vi "Write To Report.vi"(8 "error in (no error)":errorcluster, 11 "Report Info":T1[](array[typedef])) -> (0 "error out":errorcluster)   [LabVIEW 2018, in "File IO.lvlib"]
doc: "This subVI enqueues the named action in to the communications queue along with the input data."
uses:
  File IO.lvlib
  Private Controls/Module Action.ctl
  Public Controls/Write to Report.ctl
  Public Controls/Report Sheet Names.ctl
  Private Controls/Module Data.ctl
panel:
  in  "Action":T3=enum."Write To Report"
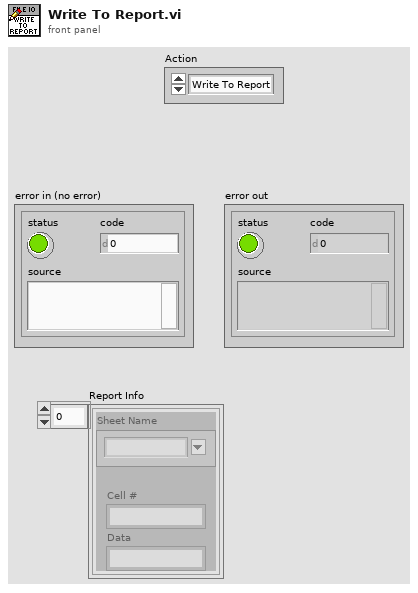
[diagram p1: front panel]
types:
  T1 = typedef "File IO.lvlib/Write to Report.ctl" = cluster{"Sheet Name":T2, "Cell #":string, "Data":string}
  T2 = typedef "File IO.lvlib/Report Sheet Names.ctl" = string
  T3 = typedef "File IO.lvlib/Module Action.ctl" = enum8{"Timeout", "OpenReport", "Continue Test", "Init", "Error", "Exit", "Save Accel Data", "Set Recording State", "Log APU RunTime", "Start New Test", "Create New Reports", "Write to System Log", "Save Variables", "Load APU Setup File", "Increment Run Count", "Write To Report"}
  T4 = typedef "File IO.lvlib/Module Data.ctl" = cluster{"Data":variant, "Action":T3}
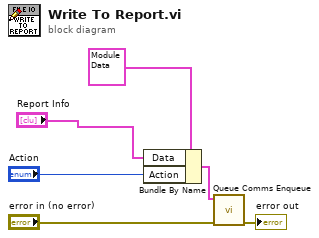
[diagram p0: block diagram]
diagram:
  n1 = Bundle By Name(cluster=T4 {"Data"=variant, "Action"=enum."Init"} ("element"), "Data"="Report Info", "Action"="Action") -> (w6:T4)
  n2 = call "Queue Comms Enqueue.vi"("error in (no error)"="error in (no error)", "element"=w6) -> ("error out"=→"error out":errorcluster)  [unwired: 9 in]
